vi "GET URI File name.vi"(11 "URI":string) -> (1 "Full Path":string[](array[string]), 2 "Is File":bool, 3 "File Name":string)   [LabVIEW 2019, in "HTTP Server.lvlib"]
uses:
  HTTP Server.lvlib
panel:
  out "匹配后偏移量":i32
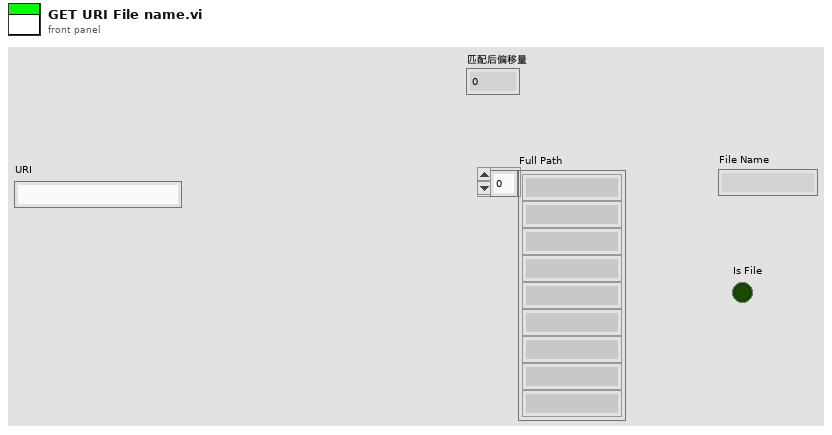
[diagram p1: front panel]
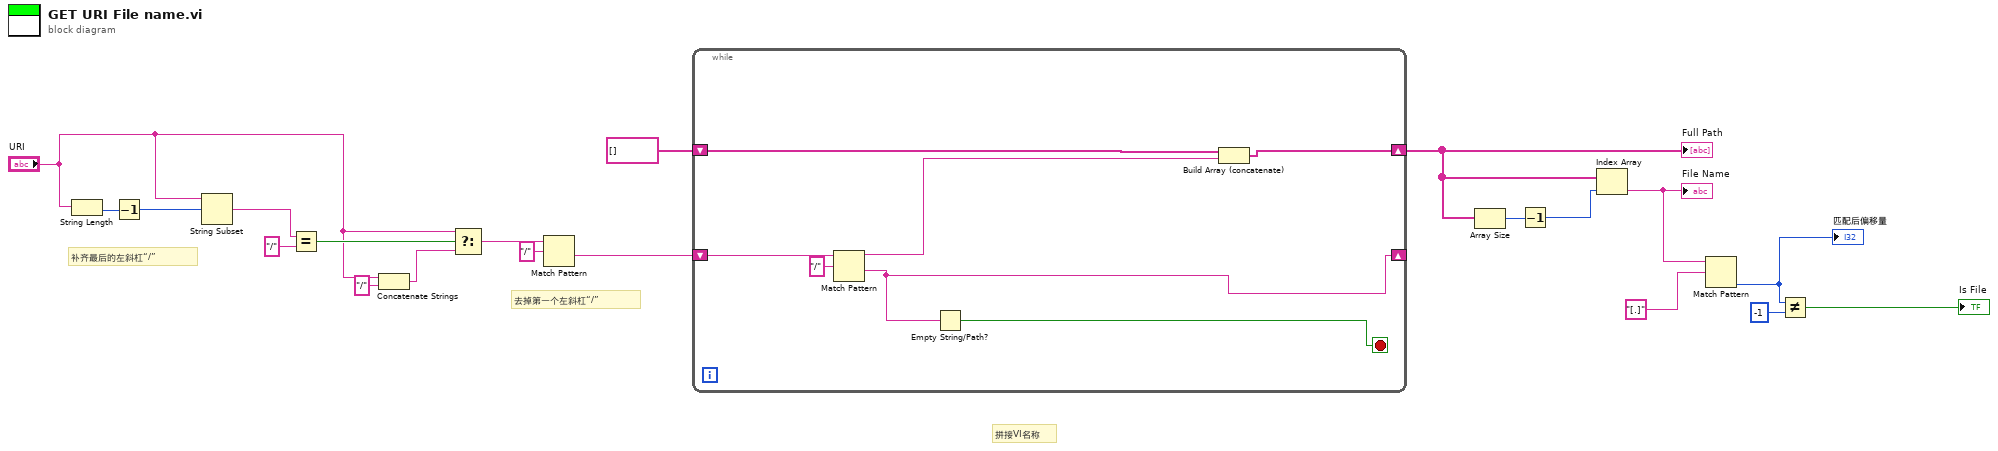
[diagram p0: block diagram]
diagram:
  # "拼接VI名称"
  # "去掉第一个左斜杠“/”"
  # "补齐最后的左斜杠“/”"
  n1 = String Length(string="URI") -> (length=w20:i32)
  n2 = Decrement(x=w20) -> (x-1=w19:i32)
  n3 = String Subset(string="URI", offset (0)=w19) -> (substring=w18:string)  [unwired: 1 in]
  n4 = Equal?(x=w18, y="/") -> (x = y?=w16:bool)
  n5 = Concatenate Strings("URI", "/" ("字符串")) -> (w14:string)
  n6 = Select(t="URI", s=w16, f=w14) -> (s? t:f=w13:string)
  n7 = Match Pattern(string=w13, regular expression="/" ("正则表达式")) -> (after substring=w11:string)  [unwired: 1 in, 3 out]
  n8 = while {
    shift-right: [w22] -> _
    shift-left: w11 -> [w25]
    shift-right: [w26] -> w1
    shift-left: string[] [] -> [w27]
    stop <- w21 stop-if-true
    n9 = Match Pattern(string=w25, regular expression="/" ("正则表达式")) -> (before substring=w23:string, after substring=w22:string)  [unwired: 1 in, 2 out]
    n10 = Empty String/Path?(string/path=w22) -> (empty?=w21:bool)
    n11 = Build Array (concatenate)(w27, w23) -> (w26:string[])
  }
  "Full Path" <- w1
  n12 = Array Size(array=w1) -> (size(s)=w8:i32)
  n13 = Decrement(x=w8) -> (x-1=w7:i32)
  n14 = Index Array(array=w1, index=w7) -> (element=w6:string)
  "File Name" <- w6
  n15 = Match Pattern(string=w6, regular expression="[.]" ("正则表达式")) -> (offset past match=w4:i32)  [unwired: 1 in, 3 out]
  "匹配后偏移量" <- w4
  n16 = Not Equal?(x=w4, y=-1) -> (x != y?=→"Is File":bool)
